vi "Matrix Fundamentals.vi"() -> ()   [LabVIEW 2023]
doc: "Shows the fundamental behavior and functionality of the matrix data type. While the test is running, you can change the matrix inputs or select built-in or user-defined numeric operations. Change the operation mode between matrix and array versions of the operations to see the difference in results."
uses:
  <vilib>/Analysis/Matrix/Datatypes/RealMatrix.ctl
  <vilib>/Analysis/Matrix/Datatypes/ComplexMatrix.ctl
  <vilib>/Analysis/Matrix/Numeric/Add/Add - RM,RM.vi
  <vilib>/Analysis/Matrix/Numeric/Conversions/Matrix To Array - RM.vi
  <vilib>/Analysis/Matrix/Numeric/Conversions/Array To Matrix - RA2.vi
  <vilib>/Analysis/Matrix/Numeric/Multiply/Multiply - RM,RM.vi
  <vilib>/Analysis/Matrix/Numeric/Exponential/Exponential - RM.vi
  <vilib>/Analysis/Matrix/Numeric/Natural Logarithm/Natural Logarithm - RM.vi
  <vilib>/Analysis/Matrix/Numeric/Square Root/Square Root - RM.vi
  <vilib>/Analysis/Matrix/Numeric/Conversions/Array To Matrix - CA2.vi
  <vilib>/Analysis/Matrix/Numeric/Complex/Cartesian To Complex - RM,RM.vi
  <vilib>/Analysis/Matrix/Numeric/Conversions/Array To Matrix - RA.vi
  <vilib>/Analysis/Matrix/NI_Matrix.lvlib
panel:
  in  "Mode":u16(ring) items=["Array", "Matrix"]
  in  "Stop":bool
  in  "Real Matrix B":T1=[[1.0, 2.0], [3.0, 4.0]]
  out "Complex Matrix Result":T2
  out "Real Matrix Result":T1
  in  "Operation":u16(ring) items=["Decrement", "Add", "Multiply", "Exponential", "Natural Logarithm", "Square Root", "Cartesian To Complex", "Add Identity", "Sum Columns"]
  in  "Real Matrix A":T1=[[1.0, 0.0], [1.0, 1.0]]
  # "Overview: Demonstrates the fundamental behavior and functionality of the Matrix data type.\nRequirements: LabVIEW Full Development System\nInstructions: \n1. Run the VI.\n2. Modify the Real Matrix inputs, Operation and Mode, and view the Real Matrix Result.\n3. Click Stop to stop the VI."
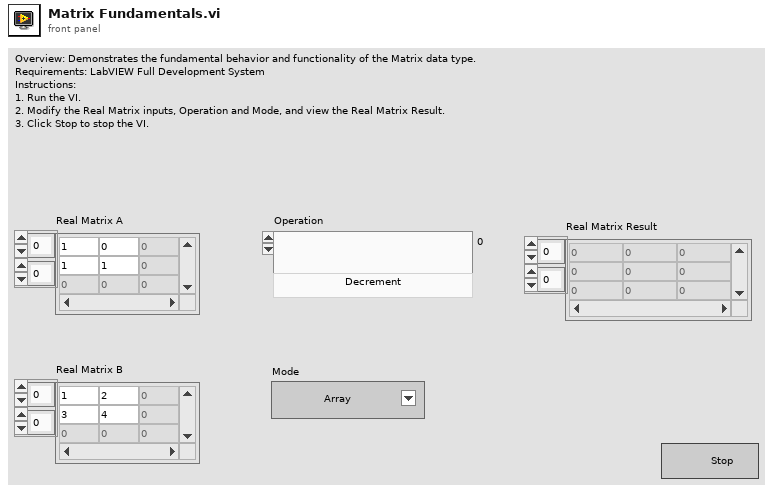
[diagram p1: front panel]
types:
  T1 = typedef "NI_Matrix.lvlib/RealMatrix.ctl" = dbl[][]
  T2 = typedef "NI_Matrix.lvlib/ComplexMatrix.ctl" = cdb[][]
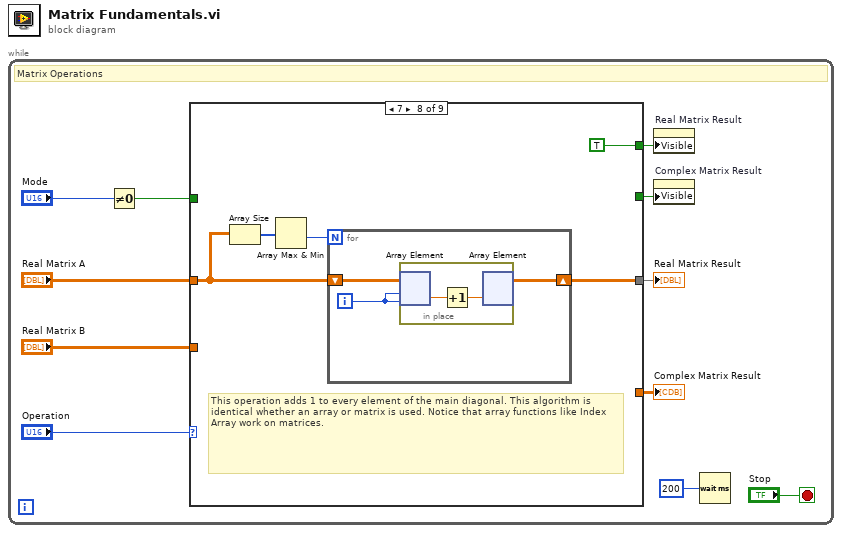
[diagram p0: block diagram]
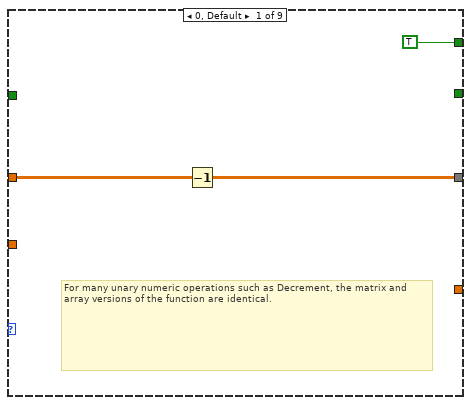
[diagram p2: hidden frame]
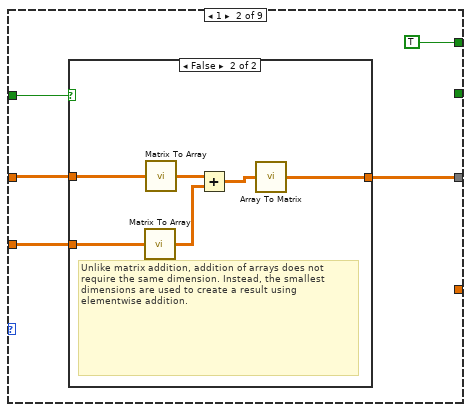
[diagram p3: hidden frame]
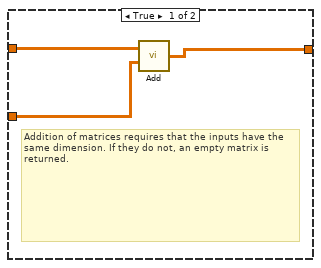
[diagram p4: hidden frame]
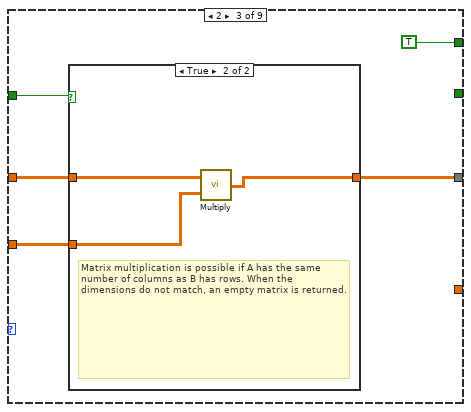
[diagram p5: hidden frame]
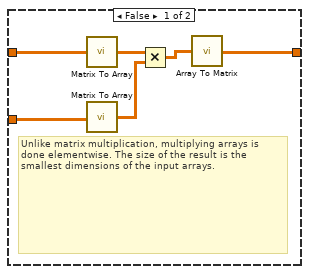
[diagram p6: hidden frame]
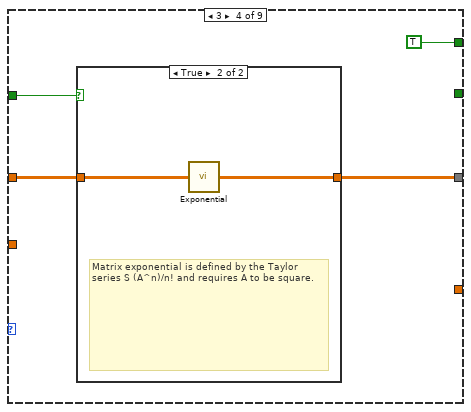
[diagram p7: hidden frame]
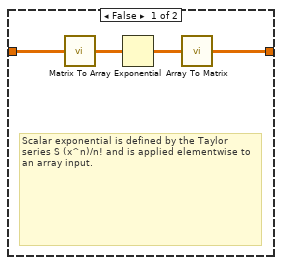
[diagram p8: hidden frame]
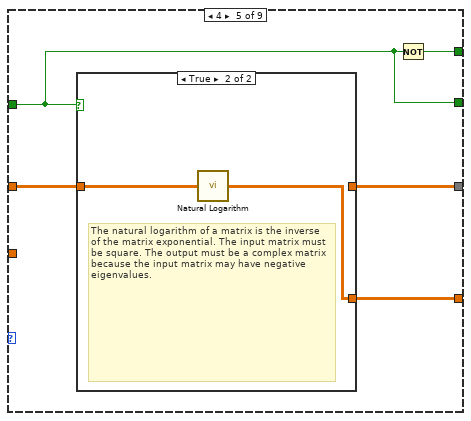
[diagram p9: hidden frame]
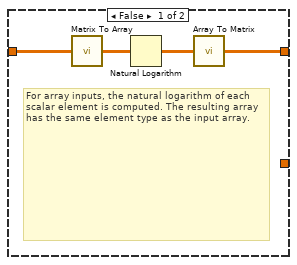
[diagram p10: hidden frame]
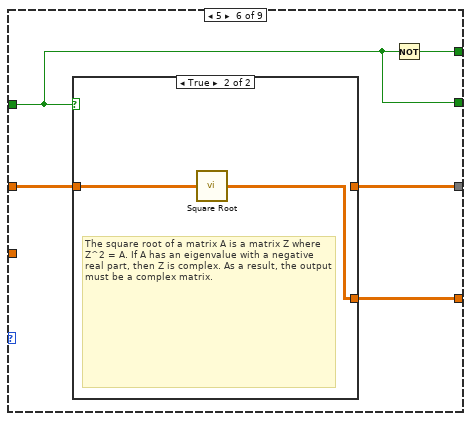
[diagram p11: hidden frame]
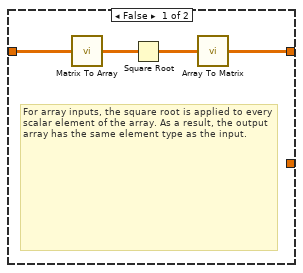
[diagram p12: hidden frame]
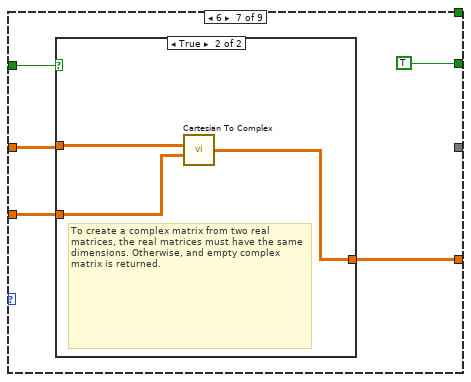
[diagram p13: hidden frame]
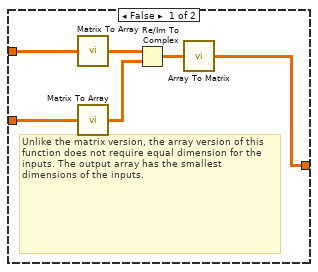
[diagram p14: hidden frame]
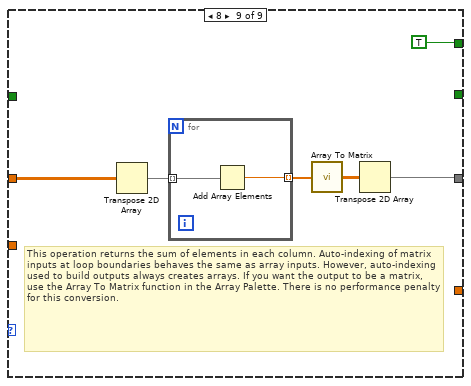
[diagram p15: hidden frame]
diagram:
  n1 = while {
    stop <- "Stop" stop-if-true
    # "Matrix Operations"
    n2 = Not Equal To 0?(x="Mode") -> (x != 0?=w1:bool)
    n3 = case shown="7" "Operation" {
      tunnel: "Real Matrix A" -> [w14 w19 w33 w45 w57 w68 w79 w91 w104]
      tunnel: [w13 w17 w31 w46 w55 w66 _ w89 w100] -> w9
      tunnel: "Real Matrix B" -> [_ w18 w32 _ _ _ w78 _ _]
      tunnel: [_ _ _ _ w56 w67 w77 _ _] -> w7
      tunnel: w1 -> [_ w16 w29 w43 w53 w64 w75 _ _]
      tunnel: [TRUE TRUE TRUE TRUE w54 w65 _ TRUE TRUE] -> w6
      tunnel: [_ _ _ _ w53 w64 TRUE _ _] -> w5
      frame 0, Default {
        # "For many unary numeric operations such as Decrement, the matrix and array versions of the function are identical."
        n4 = Decrement(x=w14) -> (x-1=w13:T1)
      }
      frame 1 {
        n5 = case shown="False" w16 {
          tunnel: w19 -> [w22 w28]
          tunnel: w18 -> [w21 w27]
          tunnel: [w20 w23] -> w17
          frame True {
            # "Addition of matrices requires that the inputs have the same dimension. If they do not, an empty matrix is returned."
            n6 = call-poly <vilib>:"Add.vi"("Real Matrix B"=w21, "Real Matrix A"=w22) -> ("A + B"=w20:T1)
          }
          frame False {
            # "Unlike matrix addition, addition of arrays does not require the same dimension. Instead, the smallest dimensions are used to create a result using elementwise addition."
            n7 = call-poly <vilib>:"Matrix To Array.vi"("Real Matrix"=w27) -> ("Real 2D Array"=w24:dbl[][])
            n8 = call-poly <vilib>:"Matrix To Array.vi"("Real Matrix"=w28) -> ("Real 2D Array"=w25:dbl[][])
            n9 = Add ("Add.vi")(x=w25, y=w24) -> (x+y=w26:dbl[][])
            n10 = call-poly <vilib>:"Array To Matrix.vi"("Real 2D Array"=w26) -> ("Real Matrix"=w23:T1)
          }
        }
      }
      frame 2 {
        n11 = case shown="True" w29 {
          tunnel: w33 -> [w36 w42]
          tunnel: w32 -> [w35 w41]
          tunnel: [w39 w40] -> w31
          frame False {
            # "Unlike matrix multiplication, multiplying arrays is done elementwise. The size of the result is the smallest dimensions of the input arrays."
            n12 = call-poly <vilib>:"Matrix To Array.vi"("Real Matrix"=w36) -> ("Real 2D Array"=w37:dbl[][])
            n13 = call-poly <vilib>:"Matrix To Array.vi"("Real Matrix"=w35) -> ("Real 2D Array"=w34:dbl[][])
            n14 = Multiply(x=w37, y=w34) -> (x*y=w38:dbl[][])
            n15 = call-poly <vilib>:"Array To Matrix.vi"("Real 2D Array"=w38) -> ("Real Matrix"=w39:T1)
          }
          frame True {
            # "Matrix multiplication is possible if A has the same number of columns as B has rows. When the dimensions do not match, an empty matrix is returned."
            n16 = call-poly <vilib>:"Multiply.vi"("Real Matrix B"=w41, "Real Matrix A"=w42) -> ("A * B"=w40:T1)
          }
        }
      }
      frame 3 {
        n17 = case shown="True" w43 {
          tunnel: [w48 w52] -> w46
          tunnel: w45 -> [w50 w51]
          frame False {
            # "Scalar exponential is defined by the Taylor series S (x^n)/n! and is applied elementwise to an array input."
            n18 = call-poly <vilib>:"Matrix To Array.vi"("Real Matrix"=w50) -> ("Real 2D Array"=w49:dbl[][])
            n19 = Exponential ("Exponential.vi")(1:w49) -> (0:w47:dbl[][])
            n20 = call-poly <vilib>:"Array To Matrix.vi"("Real 2D Array"=w47) -> ("Real Matrix"=w48:T1)
          }
          frame True {
            # "Matrix exponential is defined by the Taylor series S (A^n)/n! and requires A to be square."
            n21 = call-poly <vilib>:"Exponential.vi"("Real Matrix A"=w51) -> ("e^A"=w52:T1)
          }
        }
      }
      frame 4 {
        n22 = case shown="True" w53 {
          tunnel: w57 -> [w59 w63]
          tunnel: [_ w62] -> w56
          tunnel: [w58 _] -> w55
          frame False {
            # "For array inputs, the natural logarithm of each scalar element is computed. The resulting array has the same element type as the input array."
            n23 = call-poly <vilib>:"Matrix To Array.vi"("Real Matrix"=w59) -> ("Real 2D Array"=w60:dbl[][])
            n24 = Natural Logarithm ("Natural Logarithm.vi")(1:w60) -> (0:w61:dbl[][])
            n25 = call-poly <vilib>:"Array To Matrix.vi"("Real 2D Array"=w61) -> ("Real Matrix"=w58:T1)
          }
          frame True {
            # "The natural logarithm of a matrix is the inverse  of the matrix exponential. The input matrix must be square. The output must be a complex matrix because the input matrix may have negative eigenvalues."
            n26 = call-poly <vilib>:"Natural Logarithm.vi"("Real Matrix A"=w63) -> ("ln(A)"=w62:T2)
          }
        }
        n27 = Not(x=w53) -> (.not. x?=w54:bool)
      }
      frame 5 {
        n28 = case shown="True" w64 {
          tunnel: w68 -> [w72 w74]
          tunnel: [_ w73] -> w67
          tunnel: [w69 _] -> w66
          frame False {
            # "For array inputs, the square root is applied to every scalar element of the array. As a result, the output array has the same element type as the input."
            n29 = call-poly <vilib>:"Matrix To Array.vi"("Real Matrix"=w72) -> ("Real 2D Array"=w71:dbl[][])
            n30 = Square Root ("Square Root.vi")(x=w71) -> (sqrt(x)=w70:dbl[][])
            n31 = call-poly <vilib>:"Array To Matrix.vi"("Real 2D Array"=w70) -> ("Real Matrix"=w69:T1)
          }
          frame True {
            # "The square root of a matrix A is a matrix Z where Z^2 = A. If A has an eigenvalue with a negative real part, then Z is complex. As a result, the output must be a complex matrix."
            n32 = call-poly <vilib>:"Square Root.vi"("Real Matrix A"=w74) -> ("sqrt(A)"=w73:T2)
          }
        }
        n33 = Not(x=w64) -> (.not. x?=w65:bool)
      }
      frame 6 {
        n34 = case shown="True" w75 {
          tunnel: w79 -> [w84 w88]
          tunnel: w78 -> [w85 w87]
          tunnel: [w80 w86] -> w77
          frame False {
            # "Unlike the matrix version, the array version of this function does not require equal dimension for the inputs. The output array has the smallest dimensions of the inputs."
            n35 = call-poly <vilib>:"Matrix To Array.vi"("Real Matrix"=w84) -> ("Real 2D Array"=w83:dbl[][])
            n36 = call-poly <vilib>:"Matrix To Array.vi"("Real Matrix"=w85) -> ("Real 2D Array"=w82:dbl[][])
            n37 = Re/Im To Complex ("Cartesian To Complex.vi")(1:w82, 2:w83) -> (0:w81:cdb[][])
            n38 = call-poly <vilib>:"Array To Matrix.vi"("Complex 2D Array"=w81) -> ("Complex Matrix"=w80:T2)
          }
          frame True {
            # "To create a complex matrix from two real matrices, the real matrices must have the same dimensions. Otherwise, and empty complex matrix is returned."
            n39 = call-poly <vilib>:"Cartesian To Complex.vi"("Real Matrix I"=w87, "Real Matrix R"=w88) -> ("R + Ii"=w86:T2)
          }
        }
      }
      frame 7 {
        # "This operation adds 1 to every element of the main diagonal. This algorithm is identical whether an array or matrix is used. Notice that array functions like Index Array work on matrices."
        n40 = Array Size(array=w91) -> (size(s)=w92:i32[])
        n41 = Array Max & Min(array=w92) -> (min value=w90:i32)  [unwired: 3 out]
        n42 = for {
          N: w90 -> [_]
          shift-right: [w95] -> w89
          shift-left: w91 -> [w96]
          i -> [w94]
          n43 = in-place {
            n44 = in-place-array #1(w96, w94, w94) -> (w98:dbl)
            n45 = Increment(x=w98) -> (x+1=w97:dbl)
            n46 = in-place-array #1(w97) -> (w95:T1)  [unwired: 2 out]
          }
        }
      }
      frame 8 {
        # "This operation returns the sum of elements in each column. Auto-indexing of matrix inputs at loop boundaries behaves the same as array inputs. However, auto-indexing used to build outputs always creates arrays. If you want the output to be a matrix, use the Array To Matrix function in the Array Palette. There is no performance penalty for this conversion."
        n47 = Transpose 2D Array(2D array=w104) -> (transposed array=w103:T1)
        n48 = for {
          tunnel: w103 -> [w106] mode=indexing
          tunnel: [w105] -> w102 mode=indexing
          n49 = Add Array Elements(numeric array=w106) -> (sum=w105:dbl)
        }
        n50 = call-poly <vilib>:"Array To Matrix.vi"("Real 1D Array"=w102) -> ("Real Matrix (Column Vector)"=w101:T1)
        n51 = Transpose 2D Array(2D array=w101) -> (transposed array=w100:T1)
      }
    }
    "Real Matrix Result" <- w9
    "Complex Matrix Result" <- w7
    n52 = property on="Real Matrix Result" class="Arr (strict)"("Visible"=w6) -> ()  [unwired: 2 in, 2 out]
    n53 = property on="Complex Matrix Result" class="Arr (strict)"("Visible"=w5) -> ()  [unwired: 2 in, 2 out]
    n54 = Wait (ms)(milliseconds to wait=u32 200 ("millisecond timer value")) -> ()  [unwired: 1 out]
  }
